vi "Register Status for Client.vi"(0 "Status":string, 1 "TcpRouter-Client in":refnum<class "TcpRouter-Client.lvclass">, 9 "CSM Name":string="*", 11 "error in (no error)":errorcluster, 12 "Response Timeout(5000ms)":i32=5000) -> (4 "CSM Name(dup)":string, 15 "error out":errorcluster)   [LabVIEW 2020, in "CSM-TCP-Router.lvlib" / "TcpRouter-Client.lvclass"]
uses:
  TcpRouter-Client.lvclass
  TcpRouter-Client.lvclass/TcpRouter-Client.ctl
  _support/tcp-msg type.ctl
  5c4b9d63-4fec-4512-8845-8d145ac2895f.vi
  <userlib>/_NEVSTOP/Communicable State Machine(CSM)/AdvanceAPI/CSM - Revert Arguments-Safe String.vi
  <userlib>/_NEVSTOP/Communicable State Machine(CSM)/_Shared/Trim Single-line Text.vi
  <userlib>/_NEVSTOP/Communicable State Machine(CSM)/AdvanceAPI/CSM - Keywords.vi
  <userlib>/_NEVSTOP/Communicable State Machine(CSM)/_Polymophic/Build Register Message.vi
  <userlib>/_NEVSTOP/Communicable State Machine(CSM)/Communicable State Machine.lvlib
  CSM-TCP-Router.lvlib
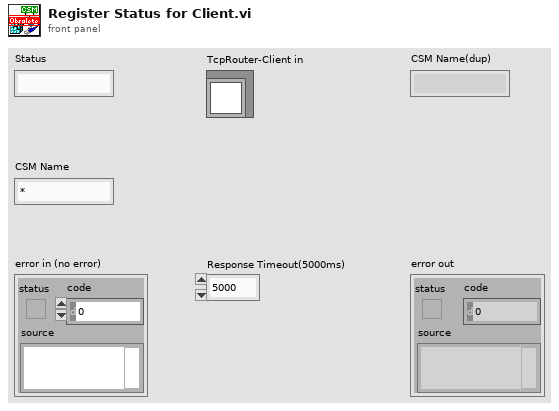
[diagram p1: front panel]
types:
  T1 = typedef "CSM-TCP-Router.lvlib/tcp-msg type.ctl" = enum8{"info", "error", "cmd", "cmd-resp", "resp", "async-resp", "status", "interrupt"}
  T2 = typedef "CSM-TCP-Router.lvlib/TcpRouter-Client.lvclass/Def-TCP-Router PUB-SUB.ctl" = cluster{"STATUS":refnum<k5>, "StatusQueue":refnum<queue>}
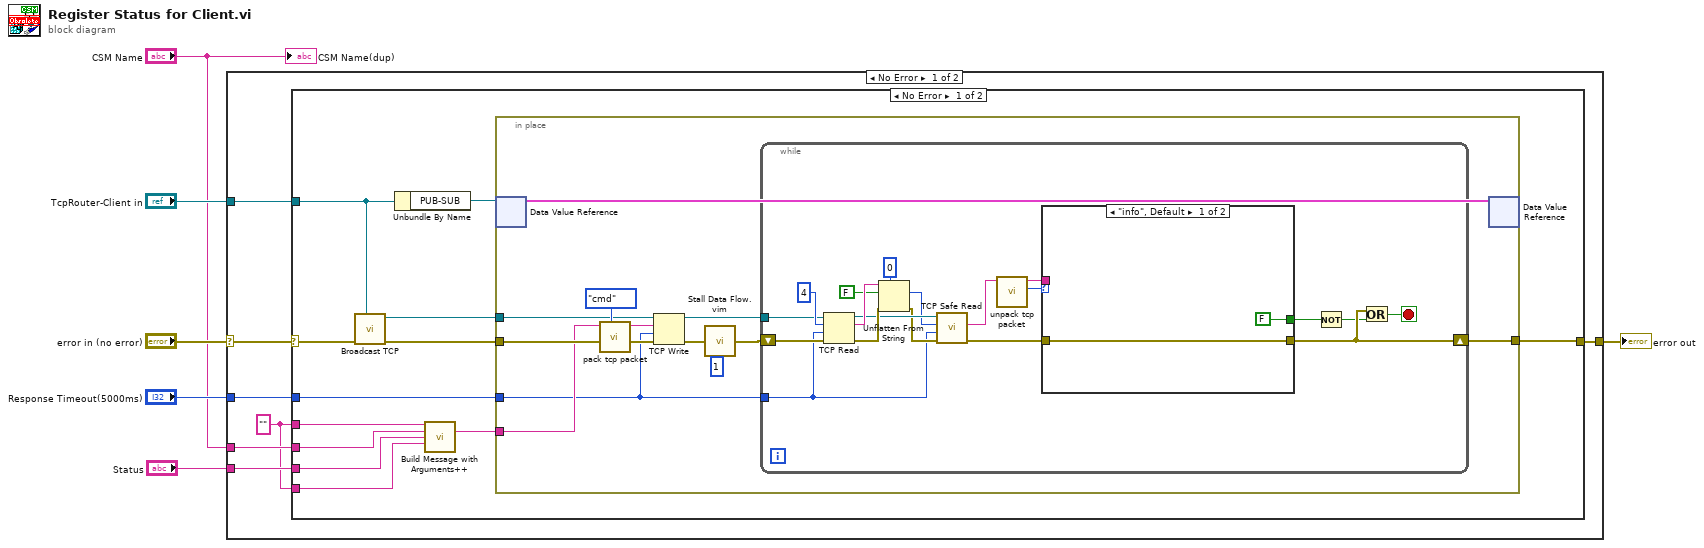
[diagram p0: block diagram]
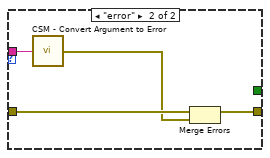
[diagram p2: hidden frame]
diagram:
  n1 = case shown="No Error" "error in (no error)" {
    selector: "error in (no error)" -> [w13 w64]
    tunnel: [w12 w64] -> w5
    tunnel: "TcpRouter-Client in" -> [w11 _]
    tunnel: "Response Timeout(5000ms)" -> [w10 _]
    tunnel: "CSM Name" -> [w9 _]
    tunnel: "Status" -> [w8 _]
    frame No Error {
      w7 = "" ("Source CSM Name (* as Default)")
      n2 = case shown="No Error" w13 {
        selector: w13 -> [w25 w63]
        tunnel: [w21 w63] -> w12
        tunnel: w11 -> [w19 _]
        tunnel: w10 -> [w20 _]
        tunnel: w7 -> [w16 _]
        tunnel: w9 -> [w17 _]
        tunnel: w8 -> [w14 _]
        tunnel: w7 -> [w15 _]
        frame No Error {
          n3 = call "Broadcast TCP.vi"("TcpRouter-Client in"=w19, "error in (no error)"=w25) -> ("error out"=w24:errorcluster, "connection ID"=w23:refnum<k5>)  [unwired: 8 in]
          n4 = Unbundle By Name(w19) -> ("PUB-SUB"=w18:refnum<data-value>)
          n5 = call-poly <userlib>:"Build Message with Arguments++.vi"("Target CSM"=w16, "Source CSM (* as Default)"=w17, "Status"=w14, "API (If \"\", Same As \"Status\")"=w15) -> ("CSM Message String"=w22:string)  [unwired: 11 in]
          n6 = in-place {
            in-place-border: w24 -> [w35]
            in-place-border: w23 -> [w34]
            in-place-border: w22 -> [w33]
            in-place-border: [w28] -> w21
            in-place-border: w20 -> [w27]
            n7 = in-place-dvr #1(w18) -> (w26:T2)  [unwired: 1 out]
            n8 = call "pack tcp packet.vi"("tcp-message-type"=tcp-msg_type."cmd", "String"=w33) -> ("TCP Pack"=w37:string)  [unwired: 9 in]
            n9 = TCP Write(connection ID=w34, data in=w37, error in (no error)=w35, 9:w27) -> (connection ID out=w30:refnum<k5>, error out=w32:errorcluster)  [unwired: 1 out]
            n10 = call "Stall Data Flow.vim"("value in"=w32, "milliseconds to wait"=u32 1) -> ("value out"=w29:errorcluster)  [unwired: 1 out]
            n11 = while {
              tunnel: w30 -> [w47]
              shift-right: [w42] -> w28
              shift-left: w29 -> [w46]
              tunnel: w27 -> [w41]
              stop <- w40 stop-if-true
              n12 = TCP Read(connection ID=w47, bytes to read=4, error in (no error)=w46, 9:w41) -> (connection ID out=w54:refnum<k5>, data out=w55:string, error out=w56:errorcluster)  [unwired: 1 in]
              n13 = Unflatten From String(type=0, binary string=w55, data includes array or string size? (T)=FALSE, error in (no error)=w56) -> (value=w52:i32, error out=w51:errorcluster)  [unwired: 2 out]
              n14 = call "TCP Safe Read.vi"("error in (no error)"=w51, "timeout ms (25000)"=w41, "bytes to read"=w52, "TCP Network Connection in"=w54) -> ("error out"=w44:errorcluster, "String"=w53:string)  [unwired: 5 in, 1 out]
              n15 = call "unpack tcp packet.vi"("TCP Pack"=w53) -> ("tcp-message-type"=w45:T1, "String"=w43:string)  [unwired: 9 in]
              n16 = case shown="\"info\", Default" w45 {
                tunnel: w44 -> [w58 w62]
                tunnel: [w58 w60] -> w42
                tunnel: w43 -> [_ w61]
                tunnel: [FALSE _] -> w39
                frame "info", Default {
                }
                frame "error" {
                  n17 = call <userlib>:"CSM - Convert Argument to Error.vi"("Argument"=w61) -> ("Error"=w59:errorcluster)  [unwired: 4 in]
                  n18 = Merge Errors(w62, w59) -> (w60:errorcluster)
                }
              }
              n19 = Not(x=w39) -> (.not. x?=w38:bool)
              n20 = Or(x=w42, y=w38) -> (x .or. y?=w40:bool)
            }
            n21 = in-place-dvr #1(w26) -> ()  [unwired: 2 out]
          }
        }
        frame Error {
        }
      }
    }
    frame Error {
    }
  }
  "error out" <- w5
  "CSM Name(dup)" <- "CSM Name"
